vi "LoadScanPanel.vi"(4 "MainProgQEvent":refnum<user-event>, 6 "MainProgQ":refnum<queue>, 8 "error in (no error)":errorcluster caption="entrée d'erreur (pas d'erreur)", 9 "ScanIndex":i32[][](array[numeric]), 11 "LoadedInst":refnum<class "BaseDevice.lvclass">[](array[class])) -> (0 "sortie d'erreur":errorcluster, 1 "PanScanFunc":string[](array[string]), 2 "PanVIs":refnum<vi>[](array[refnum]), 3 "LoadedInst Out":refnum<class "BaseDevice.lvclass">[](array[class]) caption="LoadedInst")   [LabVIEW 2019, in "BaseDevice.lvclass"]
uses:
  BaseDevice.lvclass
  BaseDevice.lvclass/BaseDevice.ctl
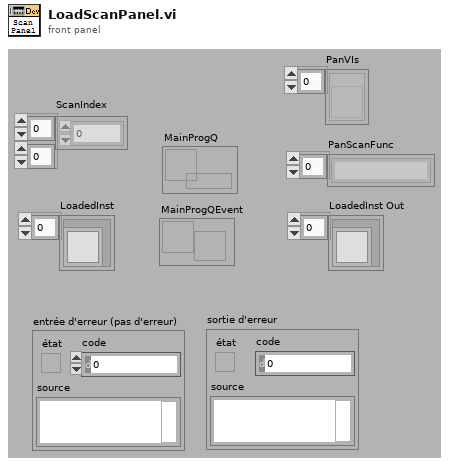
[diagram p1: front panel]
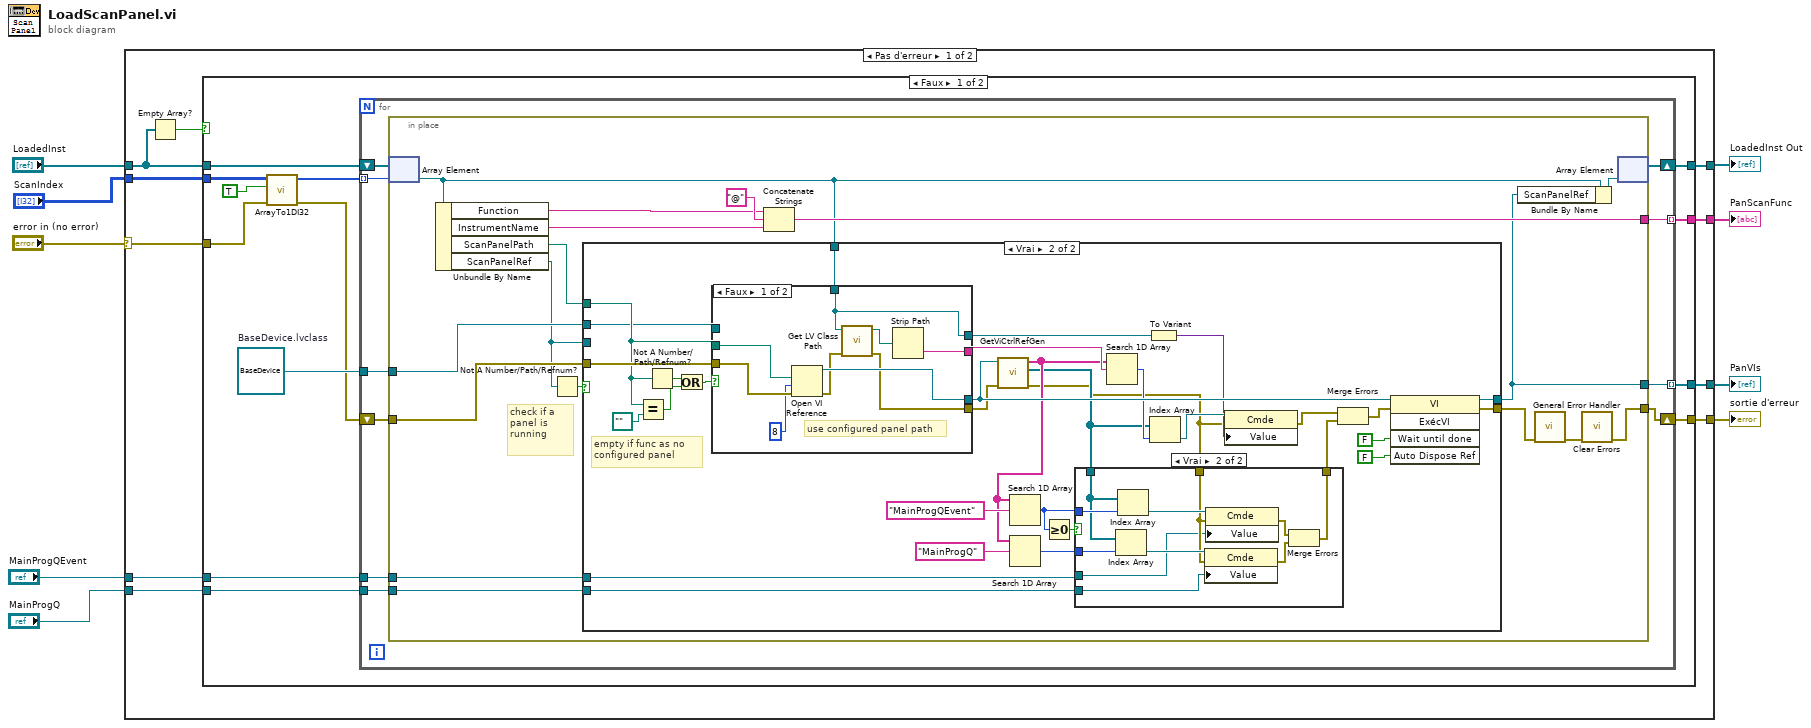
[diagram p0: block diagram]
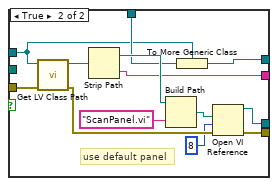
[diagram p4: hidden frame]
diagram:
  n1 = case shown="Pas d'erreur" "error in (no error)" {
    selector: "error in (no error)" -> [w15 w130]
    tunnel: [w18 w130] -> w8
    tunnel: [w19 w131] -> w6
    tunnel: "LoadedInst" -> [w14 w131]
    tunnel: "ScanIndex" -> [w12 _]
    tunnel: [w16 _] -> w5
    tunnel: [w17 _] -> w4
    tunnel: "MainProgQEvent" -> [w11 _]
    tunnel: "MainProgQ" -> [w10 _]
    frame No Error {
      n2 = Empty Array?(array=w14) -> (empty?=w13:bool)
      n3 = case shown="Faux" w13 {
        tunnel: [w32 w129] -> w19
        tunnel: [w31 w128] -> w18
        tunnel: [w29 _] -> w17
        tunnel: [w28 _] -> w16
        tunnel: w12 -> [w27 _]
        tunnel: w15 -> [w24 w128]
        tunnel: w14 -> [w23 w129]
        tunnel: w11 -> [w21 _]
        tunnel: w10 -> [w20 _]
        frame False {
          w30 = refnum<class "BaseDevice.lvclass"> refnum  # BaseDevice.lvclass
          n4 = call <userlib>:"ArrayTo1DI32.vi"("ErrorIn(No Error)"=w24, "DelArrEnd"=TRUE, "tableau"=w27) -> ("sortie d'erreur"=w26:errorcluster, "Array Out"=w25:i32[])  [unwired: 6 in, 1 out]
          n5 = for {
            shift-right: [w40] -> w32
            shift-left: w23 -> [w41]
            tunnel: w25 -> [w39] mode=indexing
            tunnel: [w38] -> w28 mode=indexing
            tunnel: [w37] -> w29 mode=indexing
            shift-right: [w42] -> w31
            shift-left: w26 -> [w36]
            tunnel: w30 -> [w35]
            tunnel: w21 -> [w34]
            tunnel: w20 -> [w33]
            n6 = in-place {
              in-place-border: w36 -> [w59]
              in-place-border: [w45] -> w42
              in-place-border: [w54] -> w38
              in-place-border: [w56] -> w37
              in-place-border: w35 -> [w51]
              in-place-border: w34 -> [w44]
              in-place-border: w33 -> [w43]
              # "check if a panel is running"
              n7 = in-place-array #1(w41, w39) -> (w47:refnum<class "BaseDevice.lvclass">)
              n8 = Unbundle By Name(w47) -> ("Function"=w52:string, "InstrumentName"=w53:string, "ScanPanelPath"=w50:path, "ScanPanelRef"=w48:refnum<vi>)
              n9 = Not A Number/Path/Refnum?(number/path/refnum=w48) -> (NaN/Path/Refnum?=w49:bool)
              n10 = case shown="Vrai" w49 {
                tunnel: w59 -> [w60 w93]
                tunnel: [w60 w90] -> w58
                tunnel: [w61 w89] -> w54
                tunnel: w51 -> [_ w81]
                tunnel: w50 -> [_ w84]
                tunnel: w48 -> [w61 _]
                tunnel: w47 -> [_ w80]
                tunnel: w44 -> [_ w63]
                tunnel: w43 -> [_ w62]
                frame False {
                  # "Panel Already running"
                }
                frame True {
                  # "empty if func as no configured panel"
                  n11 = Equal?(x=w84, y=path "") -> (x = y?=w85:bool)
                  n12 = Not A Number/Path/Refnum?(number/path/refnum=w84) -> (NaN/Path/Refnum?=w88:bool)
                  n13 = Or(x=w88, y=w85) -> (x .or. y?=w87:bool)
                  n14 = case shown="Faux" w87 {
                    tunnel: w93 -> [w114 w127]
                    tunnel: [w112 w122] -> w83
                    tunnel: [w108 w121] -> w82
                    tunnel: w84 -> [w113 _]
                    tunnel: w81 -> [_ w117]
                    tunnel: w80 -> [w106 w118]
                    tunnel: [w107 w115] -> w79
                    tunnel: [w106 w116] -> w76
                    frame False {
                      # "use configured panel path"
                      n15 = Open VI Reference(vi path=w113, options=8, error in (no error)=w114) -> (vi reference=w112:refnum<vi>, error out=w109:errorcluster)  [unwired: 3 in]
                      n16 = call <vilib>:"Get LV Class Path.vi"("error in (no error)"=w109, "object"=w106) -> ("error out"=w108:errorcluster, "class path"=w110:path)  [unwired: 8 in]
                      n17 = Strip Path(path=w110) -> (name=w107:string)  [unwired: 1 out]
                    }
                    frame True {
                      # "use default panel"
                      n18 = call <vilib>:"Get LV Class Path.vi"("error in (no error)"=w127, "object"=w117) -> ("error out"=w123:errorcluster, "class path"=w126:path)  [unwired: 8 in]
                      n19 = Strip Path(path=w126) -> (stripped path=w125:path, name=w115:string)
                      n20 = Build Path(base path=w125, name or relative path="ScanPanel.vi" ("nom ou chemin relatif")) -> (appended path=w124:path)
                      n21 = To More Generic Class(target class=w117, reference=w118) -> (generic class reference=w116:refnum<class "BaseDevice.lvclass">)
                      n22 = Open VI Reference(vi path=w124, options=8, error in (no error)=w123) -> (vi reference=w122:refnum<vi>, error out=w121:errorcluster)  [unwired: 3 in]
                    }
                  }
                  n23 = call <userlib>:"GetViCtrlRefGen.vi"("ErrorIn(No Error)"=w82, "VIRef"=w83) -> ("sortie d'erreur"=w67:errorcluster, "ControlsRefs"=w68:refnum<vi>[], "ControlsNames"=w69:string[])  [unwired: 7 in]
                  n24 = Search 1D Array(1D array=w69, element="MainProgQEvent" ("élément")) -> (index of element=w73:i32)  [unwired: 1 in]
                  n25 = Search 1D Array(1D array=w69, element="MainProgQ" ("élément")) -> (index of element=w71:i32)  [unwired: 1 in]
                  n26 = Greater Or Equal To 0?(x=w73) -> (x >= 0?=w74:bool)
                  n27 = case shown="Vrai" w74 {
                    tunnel: w73 -> [_ w105]
                    tunnel: w71 -> [_ w104]
                    tunnel: w68 -> [_ w103]
                    tunnel: w67 -> [w94 w100]
                    tunnel: [w94 w97] -> w64
                    tunnel: w63 -> [_ w96]
                    tunnel: w62 -> [_ w95]
                    frame False {
                    }
                    frame True {
                      n28 = Index Array(array=w103, index=w104) -> (element=w101:refnum<vi>)
                      n29 = Index Array(array=w103, index=w105) -> (element=w102:refnum<vi>)
                      n30 = property class="Cmde"(reference=w101, error in=w100, "Value"=w95) -> (error out=w98:errorcluster)  [unwired: 1 out]
                      n31 = property class="Cmde"(reference=w102, error in=w100, "Value"=w96) -> (error out=w99:errorcluster)  [unwired: 1 out]
                      n32 = Merge Errors(w99, w98) -> (w97:errorcluster)
                    }
                  }
                  n33 = Search 1D Array(1D array=w69, element=w79) -> (index of element=w78:i32)  [unwired: 1 in]
                  n34 = To Variant(anything=w76) -> (Variant=w75:variant)
                  n35 = Index Array(array=w68, index=w78) -> (element=w77:refnum<vi>)
                  n36 = property class="Cmde"(reference=w77, error in=w67, "Value"=w75) -> (error out=w66:errorcluster)  [unwired: 1 out]
                  n37 = Merge Errors(w66, w64) -> (w65:errorcluster)
                  n38 = invoke class="VI" method="ExécVI"(reference=w83, error in=w65, "Wait until done"=FALSE ("Attendre la fin"), "Auto Dispose Ref"=FALSE ("Supprimer la référence automatiquement")) -> (reference out=w89:refnum<vi>, error out=w90:errorcluster)  [unwired: 1 in, 3 out]
                }
              }
              n39 = Concatenate Strings(w52, "@", w53) -> (w56:string)
              n40 = Bundle By Name(cluster=w47, "ScanPanelRef"=w54) -> (w55:refnum<class "BaseDevice.lvclass">)
              n41 = call <vilib>:"General Error Handler.vi"("error in (no error)"=w58) -> ("error out"=w46:errorcluster)  [unwired: 10 in, 4 out]
              n42 = call <vilib>:"Clear Errors.vi"("error in (no error)"=w46) -> ("error out"=w45:errorcluster)  [unwired: 5 in, 1 out]
              n43 = in-place-array #1(w55) -> (w40:refnum<class "BaseDevice.lvclass">[])  [unwired: 1 out]
            }
          }
        }
        frame True {
        }
      }
    }
    frame Error {
    }
  }
  "sortie d'erreur" <- w8
  "LoadedInst Out" <- w6
  "PanVIs" <- w5
  "PanScanFunc" <- w4
